vi "VI-Change Control Data Type.vi"(0 "Control in":refnum<vi>, 7 "Data Type":variant, 11 "error in (no error)":errorcluster) -> (15 "error out":errorcluster)   [LabVIEW 2015]
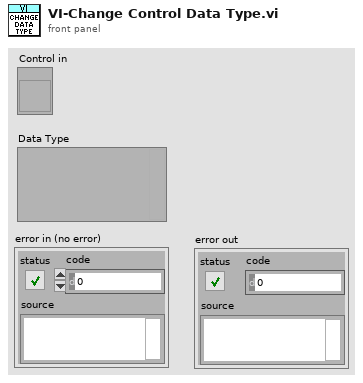
[diagram p1: front panel]
types:
  T1 = enum8{"Probe", "Diagram", "Panel Control", "3D Panel Control", "Dialog Panel Control", "Panel Indicator", "3D Panel Indicator", "Dialog Panel Indicator", "Power PC Control", "Power PC Indicator", "Silver Control", "Silver Indicator"}
  T2 = enum32{"invalid VI type", "Standard VI", "Control VI", "Global VI", "Polymorphic VI", "Configuration VI", "SubSystem", "Facade VI", "Method VI", "Statechart Diagram VI"}
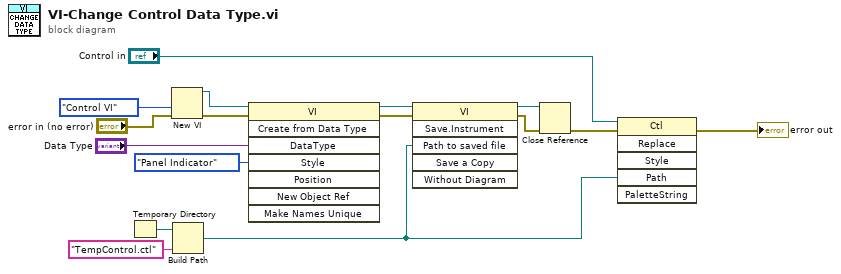
[diagram p0: block diagram]
diagram:
  n1 = Temporary Directory() -> (w8:path)
  n2 = New VI(8:"error in (no error)", 9:T2."Control VI" ("vi type (standard vi)")) -> (0:w4:errorcluster, 3:w3:refnum<vi>)  [unwired: 5 in]
  n3 = Build Path(base path=w8, name or relative path="TempControl.ctl") -> (appended path=w13:path)
  n4 = invoke class="VI" method="Create from Data Type"(reference=w3, error in=w4, "DataType"="Data Type", "Style"=T1."Panel Indicator") -> (reference out=w6:refnum<vi>, error out=w7:errorcluster)  [unwired: 4 in, 6 out]
  n5 = invoke class="VI" method="Save.Instrument"(reference=w6, error in=w7, "Path to saved file"=w13) -> (reference out=w10:refnum<vi>, error out=w11:errorcluster)  [unwired: 3 in, 4 out]
  n6 = Close Reference(reference=w10, error in (no error)=w11) -> (error out=w12:errorcluster)
  n7 = invoke class="Ctl" method="Replace"(reference="Control in", error in=w12, "Path"=w13) -> (error out=→"error out":errorcluster)  [unwired: 3 in, 5 out]
